vi "addCategory.vi"(8 "error in (no error)":errorcluster, 10 "Category.lvclass":refnum<class "Category.lvclass">, 11 "CategoryList in":refnum<class "CategoryList.lvclass">) -> (0 "error out":errorcluster, 3 "CategoryList out":refnum<class "CategoryList.lvclass">)   [LabVIEW 2018, in "CategoryList.lvclass"]
uses:
  CategoryList.lvclass
  Category/Category.lvclass
  CategoryList.lvclass/CategoryList.ctl
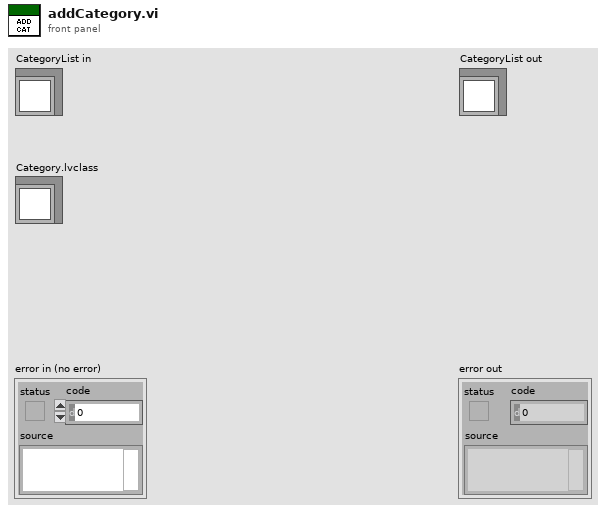
[diagram p1: front panel]
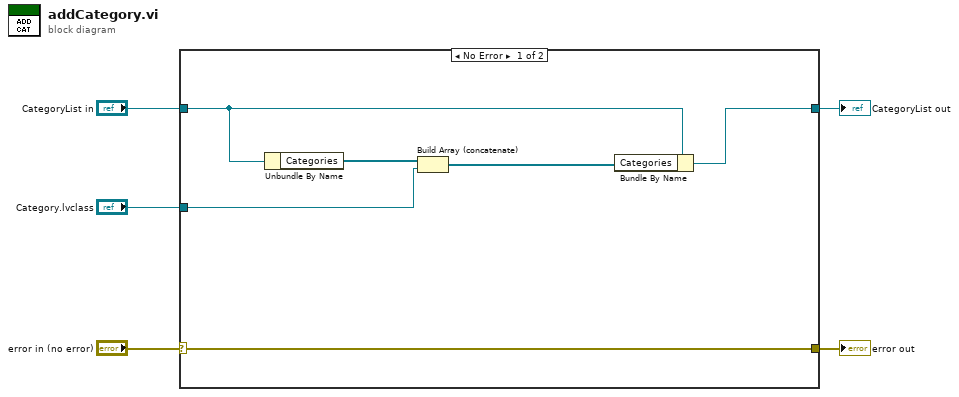
[diagram p0: block diagram]
diagram:
  n1 = case shown="No Error" "error in (no error)" {
    selector: "error in (no error)" -> [w11 w13]
    tunnel: [w11 w13] -> w4
    tunnel: [w10 w12] -> w2
    tunnel: "CategoryList in" -> [w9 w12]
    tunnel: "Category.lvclass" -> [w6 _]
    frame No Error {
      n2 = Unbundle By Name(w9) -> ("Categories"=w8:refnum<class "Category.lvclass">[])
      n3 = Build Array (concatenate)(w8, w6) -> (w7:refnum<class "Category.lvclass">[])
      n4 = Bundle By Name(cluster=w9, "Categories"=w7) -> (w10:refnum<class "CategoryList.lvclass">)
    }
    frame Error {
    }
  }
  "error out" <- w4
  "CategoryList out" <- w2
